vi "Initialize.vi"(8 "error in":errorcluster, 11 "custom device ref":T1 format="%.0x") -> (0 "error out":errorcluster, 3 "custom device ref out":T1 format="%.0x")   [LabVIEW 2020, in "AIM MIL-STD-1553 System Explorer.lvlib" / "Implementation.lvlib"]
doc: "Called by Initialization VI on launch of the custom device. Adds Configuration File and Logging sections to the custom device."
uses:
  Implementation.lvlib
  <vilib>/NI VeriStand/Custom Device API/Custom Device Item Ref.ctl
  Shared/AIM Hardware Parameters.ctl
  Shared/Initialization Method.ctl
  Shared/Bus Selection.ctl
  Shared/Coupling Mode.ctl
  Scripting/AIM MIL-STD-1553 Scripting.lvlib
  <vilib>/NI VeriStand/Custom Device API/Custom Device API.lvlib
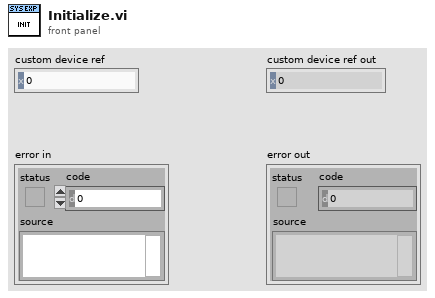
[diagram p1: front panel]
types:
  T1 = typedef "Custom Device API.lvlib/Custom Device Item Ref.ctl" = u64
  T2 = typedef "AIM Hardware Parameters.ctl" = cluster{"initialization method":T3, "card number":i32, "pxi slot number":i32, "biu number":i32, "bus selection":T4, "coupling mode":T5}
  T3 = typedef "Initialization Method.ctl" = enum16{"PXI Slot Number", "Card Number"}
  T4 = typedef "Bus Selection.ctl" = enum16{"Both", "Primary", "Secondary"}
  T5 = typedef "Coupling Mode.ctl" = enum16{"Isolated Onboard Termination", "Transformer Coupled", "Direct Coupled", "External with Onboard Termination", "Onboard Digital Wrap-around"}
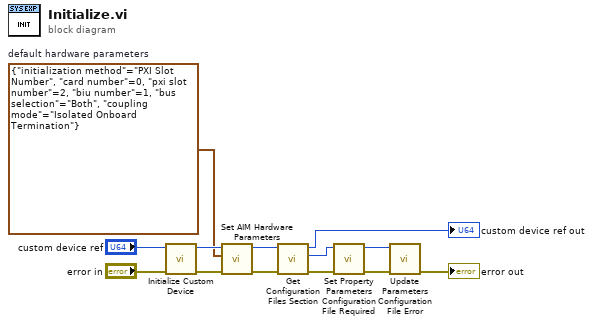
[diagram p0: block diagram]
diagram:
  w9 = T2 {"initialization method"=enum."PXI Slot Number", "card number"=0, "pxi slot number"=2, "biu number"=1, "bus selection"=enum."Both", "coupling mode"=enum."Isolated Onboard Termination"}  # default hardware parameters
  n1 = call "Initialize Custom Device.vi"("error in"="error in", "custom device ref"="custom device ref") -> ("error out"=w11:errorcluster, "custom device ref out"=w10:T1)  [unwired: 8 in]
  n2 = call "Set AIM Hardware Parameters.vi"("error in"=w11, "device parameters"=w9, "custom device ref"=w10) -> ("error out"=w7:errorcluster, "custom device ref out"=w8:T1)  [unwired: 7 in]
  n3 = call "Get Configuration Files Section.vi"("error in"=w7, "custom device in"=w8) -> ("error out"=w4:errorcluster, "configuration files section"=w5:T1, "custom device out"=→"custom device ref out":T1)  [unwired: 6 in, 1 out]
  n4 = call "Set Property Parameters Configuration File Required.vi"("error in"=w4, "configuration files ref"=w5) -> ("error out"=w2:errorcluster, "configuration files ref out"=w3:T1)  [unwired: 8 in]
  n5 = call "Update Parameters Configuration File Error.vi"("error in"=w2, "configuration files ref in"=w3) -> ("error out"=→"error out":errorcluster)  [unwired: 8 in, 1 out]
